vi "Express read current voltage charge.vi"(10 "Previous time":dbl, 11 "Initial time":timestamp) -> (0 "Charge (mC)":dbl, 1 "Electrolysis current (mA)":dbl, 2 "Electrolysis voltage (V)":dbl, 3 "Time (s)":dbl)   [LabVIEW 2017]
panel:
  out "delta charge (mC)":dbl
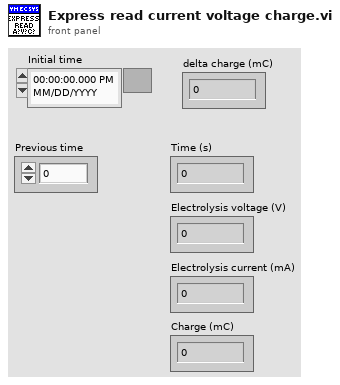
[diagram p1: front panel]
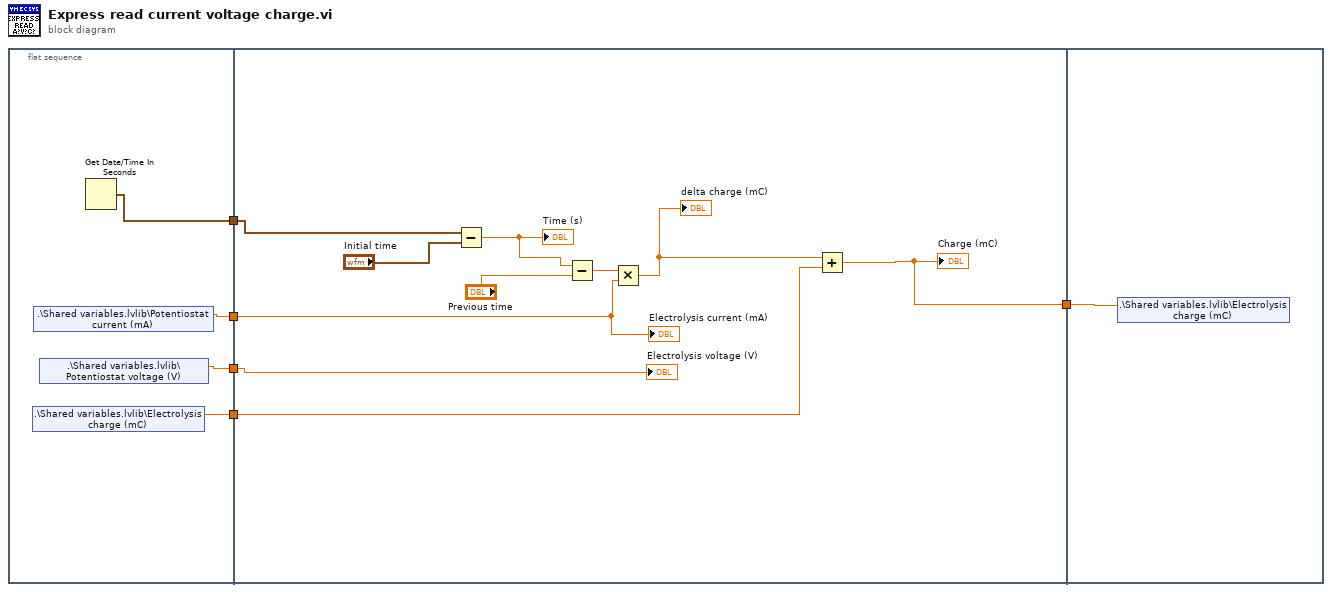
[diagram p0: block diagram]
diagram:
  n1 = flat-sequence {
    tunnel: [w9] -> w5
    tunnel: [w8] -> w4
    tunnel: [w7] -> w3
    tunnel: [w6] -> w2
    tunnel: w5 -> [w12]
    tunnel: w4 -> [w13]
    tunnel: w3 -> [w14]
    tunnel: w2 -> [w11]
    tunnel: [w10] -> w1
    tunnel: w1 -> [w20]
    frame #0 {
      n2 = shared-variable ".\\Shared variables.lvlib\\Electrolysis charge (mC)"() -> (w6:dbl)  [unwired: 1 in, 1 out]
      n3 = shared-variable ".\\Shared variables.lvlib\\Potentiostat current (mA)"() -> (w8:dbl)  [unwired: 1 in, 1 out]
      n4 = shared-variable ".\\Shared variables.lvlib\\Potentiostat voltage (V)"() -> (w9:dbl)  [unwired: 1 in, 1 out]
      n5 = Get Date/Time In Seconds() -> (seconds since 1Jan1904=w7:timestamp)
    }
    frame #1 {
      n6 = Subtract(x=w14, y="Initial time") -> (x-y=w16:dbl)
      "Time (s)" <- w16
      n7 = Subtract(x=w16, y="Previous time") -> (x-y=w18:dbl)
      n8 = Multiply(x=w18, y=w13) -> (x*y=w19:dbl)
      "delta charge (mC)" <- w19
      n9 = Add(x=w19, y=w11) -> (x+y=w10:dbl)
      "Charge (mC)" <- w10
      "Electrolysis voltage (V)" <- w12
      "Electrolysis current (mA)" <- w13
    }
    frame #2 {
      n10 = shared-variable ".\\Shared variables.lvlib\\Electrolysis charge (mC)"(w20) -> ()  [unwired: 1 in, 1 out]
    }
  }
